vi "EstimateTargetingInformation.vi"(0 "X (in) [t0]":dbl, 5 "Y (in) [t0]":dbl, 7 "Robot Heading (deg)":dbl, 12 "Acceptable Heading Error (deg)":dbl, 13 "Min Timed Aligned (ms)":u32) -> (4 "Pointed At Target":bool, 6 "Heading to Target (deg)":dbl, 8 "Distance to Target (in)":dbl, 15 "Targeting Information":dbl[](array[numeric]))   [LabVIEW 2023]
doc: "This VI estimates the robot's heading and distance to the nearest requested scoring location."
uses:
  <vilib>/Rock Robotics/WPI/DriverStation/WPI_DriverStationAllianceInfo.ctl
  GlobalDriverStationData.vi
  GlobalPoseAndTargeting.vi
  GlobalDriverStationCommands.vi
  GlobalDrivebase.vi
panel:
  in  "OUT_Scoring_Position":T1(ring)
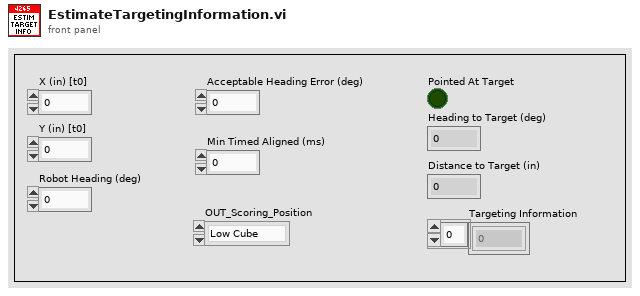
[diagram p1: front panel]
types:
  T1 = enum16{"Low Cube", "Mid Cube", "High Cube", "Low Cone", "Mid Cone", "High Cone"}
  T2 = typedef "WPI_DriverStationAllianceInfo.ctl" = enum16{"Red", "Blue", "Invalid"}
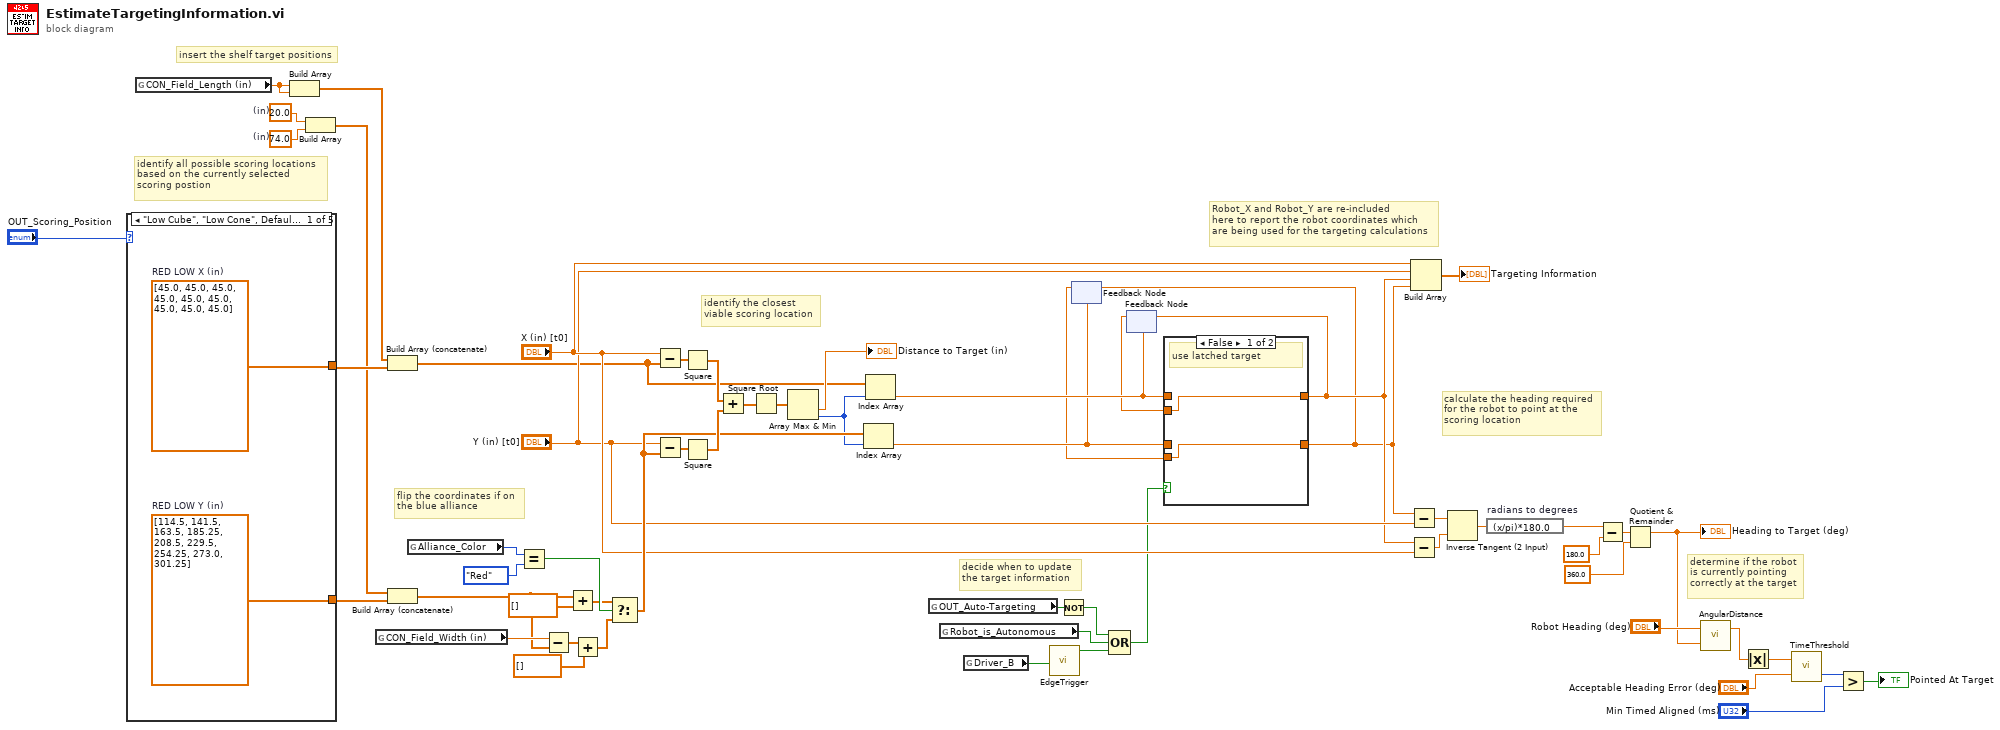
[diagram p0: block diagram]
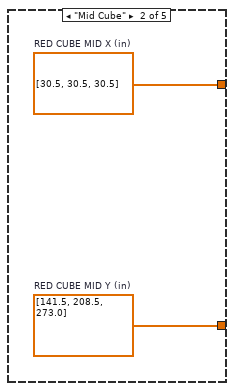
[diagram p3: hidden frame]
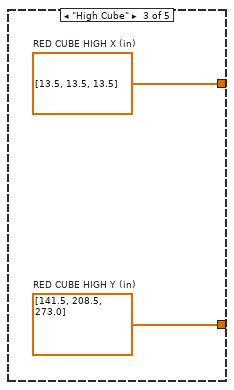
[diagram p4: hidden frame]
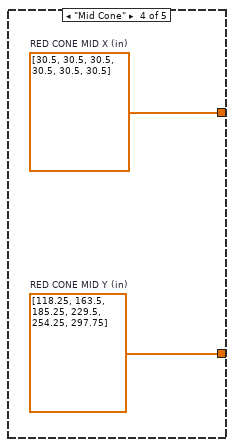
[diagram p5: hidden frame]
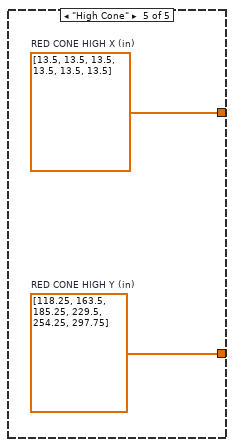
[diagram p6: hidden frame]
diagram:
  w4 = 20.0  # (in)
  w6 = 74.0  # (in)
  # "insert the shelf target positions"
  # "decide when to update\nthe target information"
  # "Robot_X and Robot_Y are re-included\nhere to report the robot coordinates which\nare being used for the targeting calculations"
  # "determine if the robot\nis currently pointing\ncorrectly at the target"
  # "calculate the heading required\nfor the robot to point at the\nscoring location"
  # "identify the closest\nviable scoring location"
  # "flip the coordinates if on\nthe blue alliance"
  # "identify all possible scoring locations\nbased on the currently selected\nscoring postion"
  n1 = case shown="\"Low Cube\", \"Low Cone\", Default" "OUT_Scoring_Position" {
    tunnel: [w60 w62 w64 w66 w68] -> w10
    tunnel: [w59 w61 w63 w65 w67] -> w12
    frame "Low Cube", "Low Cone", Default {
      w59 = dbl[] [114.5, 141.5, 163.5, 185.25, 208.5, 229.5, 254.25, 273.0, 301.25]  # RED LOW Y (in)
      w60 = dbl[] [45.0, 45.0, 45.0, 45.0, 45.0, 45.0, 45.0, 45.0, 45.0]  # RED LOW X (in)
    }
    frame "Mid Cube" {
      w61 = dbl[] [141.5, 208.5, 273.0]  # RED CUBE MID Y (in)
      w62 = dbl[] [30.5, 30.5, 30.5]  # RED CUBE MID X (in)
    }
    frame "High Cube" {
      w63 = dbl[] [141.5, 208.5, 273.0]  # RED CUBE HIGH Y (in)
      w64 = dbl[] [13.5, 13.5, 13.5]  # RED CUBE HIGH X (in)
    }
    frame "Mid Cone" {
      w65 = dbl[] [118.25, 163.5, 185.25, 229.5, 254.25, 297.75]  # RED CONE MID Y (in)
      w66 = dbl[] [30.5, 30.5, 30.5, 30.5, 30.5, 30.5]  # RED CONE MID X (in)
    }
    frame "High Cone" {
      w67 = dbl[] [118.25, 163.5, 185.25, 229.5, 254.25, 297.75]  # RED CONE HIGH Y (in)
      w68 = dbl[] [13.5, 13.5, 13.5, 13.5, 13.5, 13.5]  # RED CONE HIGH X (in)
    }
  }
  n2 = global read "GlobalPoseAndTargeting.vi" "CON_Field_Length (in)"() -> (w8:dbl)
  n3 = Build Array(w8, w8) -> (w7:dbl[])
  n4 = Build Array(w4, w6) -> (w5:dbl[])
  n5 = global read "GlobalPoseAndTargeting.vi" "CON_Field_Width (in)"() -> (w53:dbl)
  n6 = Build Array (concatenate)(w7, w10) -> (w9:dbl[])
  n7 = Build Array (concatenate)(w5, w12) -> (w11:dbl[])
  n8 = global read "GlobalDriverStationData.vi" "Alliance_Color"() -> (w57:T2)
  n9 = Equal?(x=w57, y=WPI_DriverStationAllianceInfo."Red") -> (x = y?=w55:bool)
  n10 = Subtract(x=w53, y=w11) -> (x-y=w54:dbl[])
  n11 = Add(x=w11, y=dbl[] []) -> (x+y=w25:dbl[])
  n12 = Add(x=w54, y=dbl[] []) -> (x+y=w26:dbl[])
  n13 = Select(t=w25, s=w55, f=w26) -> (s? t:f=w45:dbl[])
  n14 = Subtract(x="X (in) [t0]", y=w9) -> (x-y=w52:dbl[])
  n15 = Subtract(x="Y (in) [t0]", y=w45) -> (x-y=w51:dbl[])
  n16 = Square(x=w52) -> (x^2=w50:dbl[])
  n17 = Square(x=w51) -> (x^2=w49:dbl[])
  n18 = Add(x=w50, y=w49) -> (x+y=w48:dbl[])
  n19 = Square Root(x=w48) -> (sqrt(x)=w47:dbl[])
  n20 = Array Max & Min(array=w47) -> (min value=→"Distance to Target (in)":dbl, min index (indices)=w44:i32)  [unwired: 2 out]
  n21 = Index Array(array=w45, index=w44) -> (element=w21:dbl)
  n22 = Index Array(array=w9, index=w44) -> (element=w23:dbl)
  n23 = global read "GlobalDrivebase.vi" "OUT_Auto-Targeting"() -> (w13:bool)
  n24 = global read "GlobalDriverStationData.vi" "Robot_is_Autonomous"() -> (w15:bool)
  n25 = global read "GlobalDriverStationCommands.vi" "Driver_B"() -> (w18:bool)
  n26 = call "EdgeTrigger.vi"("Input Signal"=w18) -> ("Rising Edge Trigger"=w16:bool)  [unwired: 2 out]
  n27 = Not(x=w13) -> (.not. x?=w14:bool)
  n28 = feedback #1(w21) -> (w19:dbl)
  n29 = Compound Arithmetic op=OR(w14, w15, w16) -> (w17:bool)
  n30 = feedback #2(w23) -> (w22:dbl)
  n31 = case shown="False" w17 {
    tunnel: w23 -> [_ w72]
    tunnel: w21 -> [_ w71]
    tunnel: [w70 w72] -> w24
    tunnel: [w69 w71] -> w20
    tunnel: w22 -> [w70 _]
    tunnel: w19 -> [w69 _]
    frame False {
      # "use latched target"
    }
    frame True {
      # "update target"
    }
  }
  n32 = feedback-in #1(w20) -> ()
  n33 = feedback-in #2(w24) -> ()
  n34 = Subtract(x=w20, y="Y (in) [t0]") -> (x-y=w42:dbl)
  n35 = Subtract(x=w24, y="X (in) [t0]") -> (x-y=w41:dbl)
  n36 = Build Array("X (in) [t0]", "Y (in) [t0]", w24, w20) -> (→"Targeting Information":dbl[])
  n37 = Inverse Tangent (2 Input)(1:w41, 2:w42) -> (0:w43:dbl)
  n38 = expression code="(x/pi)*180.0" "radians to degrees"(w43) -> (w30:dbl)
  n39 = Subtract(x=w30, y=180.0) -> (x-y=w29:dbl)
  n40 = Quotient & Remainder(x=w29, y=360.0) -> (x-y*floor(x/y)=w27:dbl)  [unwired: 1 out]
  "Heading to Target (deg)" <- w27
  n41 = call "AngularDistance.vi"("Goal Angle (deg) [0,360]"=w27, "Current Angle (deg) [-Inf,+Inf]"="Robot Heading (deg)") -> ("Signed Angular Distance (deg) [-180,+180]"=w37:dbl)  [unwired: 1 out]
  n42 = Absolute Value(x=w37) -> (abs(x)=w35:dbl)
  n43 = call "TimeThreshold.vi"("Threshold"="Acceptable Heading Error (deg)", "Current Value"=w35) -> ("Time Below Threshold (ms)"=w34:u32)  [unwired: 1 out]
  n44 = Greater?(x=w34, y="Min Timed Aligned (ms)") -> (0:→"Pointed At Target":bool)
